vi "main.vi"() -> ()   [LabVIEW 2020]
uses:
  <vilib>/Instr/_visa.llb/VISA Set IO Buffer Mask.ctl
  95f16878-fea6-4ba9-9ba1-5f26283d1fdc.vi
  5cf80d48-7aba-4c71-a3e5-f596ea732e1f.vi
  <vilib>/Instr/_visa.llb/VISA Configure Serial Port (Instr).vi
panel:
  in  "选项卡控件":enum32{"选项卡 1"}(tab)
  in  "?":enum32{"选项卡 1", "选项卡 2"}(tab)
  in  "退出程序":bool
  in  "开始测试":bool
  in  "?":enum32{"Init", "Config"}(tab)
  out "布尔":bool
  in  "打开设备":bool caption="元素入队列"
  in  "Kipcrle":refnum<k15> caption="resource name"
  in  "交流电压输出":dbl caption="Voltage Level"
  in  "输出模式选择":i32(ring) caption="Mode (AC Only)" items=["AC Only", "DC Only", "AC DC"]
  in  "直流偏置":dbl caption="VoltageOffset"
  in  "交流频率":dbl(ring)=50.0 caption="Frequency" items=["50HZ"=50.0, "90HZ"=90.0]
  in  "输出":bool
  in  "电压短时中断测试":bool
  in  "电源适应性测试":bool
  in  "模式选择":enum32{"随机模式"}(tab)
  in  "工作频率随机":bool
  in  "交流电压随机":bool
  in  "短时输出时间随机":bool
  in  "间隔中断时间随机":bool
  in  "关断时间随机":bool
  in  "工作电压":dbl caption="Acv"
  in  "直流偏置编程":dbl caption="Dcv"
  in  "关断电压":dbl caption="Acv"
  in  "upper bound (100)":dbl=100.0 caption="上限(V)"
  in  "lower bound (0)":dbl caption="下限(V)"
  in  "关断电压随机":bool
  in  "中断电压":dbl
  in  "t_off":dbl
  in  "t_gap":dbl
  in  "t_check":dbl
  in  "upper bound (100) 2":dbl=100.0 caption="上限(s)"
  in  "lower bound (0) 2":dbl caption="下限(s)"
  in  "t_on":dbl
  in  "upper bound (100) 3":dbl=100.0 caption="上限(s)"
  in  "lower bound (0) 3":dbl caption="下限(s)"
  in  "间隔中断电压随机":bool
  in  "lower bound (0) 4":dbl caption="下限(s)"
  in  "upper bound (100) 4":dbl=100.0 caption="上限(s)"
  in  "upper bound (100) 5":dbl=100.0 caption="上限(s)"
  in  "lower bound (0) 5":dbl caption="下限(s)"
  in  "工作频率":dbl(ring)=50.0 items=["50Hz"=50.0, "90Hz"=90.0]
  in  "upper bound (100) 6":dbl=100.0 caption="上限(100)"
  in  "lower bound (0) 6":dbl caption="下限(0)"
  in  "lower bound (0) 7":dbl caption="下限(0)"
  in  "upper bound (100) 7":dbl=100.0 caption="上限(100)"
  out "KipcrleErrorOut":errorcluster caption="error out" {"code" format="%.0x"}
  in  "?":enum32{"选项卡 1"}(tab)
  in  "单功能验证":bool
  in  "统一指令集":T1
  in  "设备数量":i8 min=0 max=2
  in  "是否通过串口检测":bool
  in  "?":enum32{"USB", "网口"}(tab)
  in  "VISA资源名称1":refnum<visa-resource-name>
  in  "VISA资源名称":refnum<visa-resource-name>
  in  "stop bits (10: 1 bit)":u16(ring)=10 caption="停止位（10: 1位）" items=["1.0"=10, "1.5"=15, "2.0"=20]
  in  "baud rate (9600)":u32=9600 caption="波特率(9600)"
  in  "parity (0:none)":enum16{"None", "Odd", "Even", "Mark", "Space"}(ring) caption="奇偶（0:无）"
  in  "baud rate (9600) 2":u32=9600 caption="波特率(9600)"
  in  "parity (0:none) 2":enum16{"None", "Odd", "Even", "Mark", "Space"}(ring) caption="奇偶（0:无）"
  in  "stop bits (10: 1 bit) 2":u16(ring)=10 caption="停止位（10: 1位）" items=["1.0"=10, "1.5"=15, "2.0"=20]
  in  "读取的字节":i32=500
  in  "远程端口或服务名称":u16
  in  "地址":string
  in  "发送":bool
  out "码词":string
  in  "自定义输入":string="~\u00010000@SCNTRG1;\u0003"
  in  "等待检测时间(s)":dbl
  out "COM1提示灯":bool
  out "布尔 2":bool
  out "错误输出":errorcluster
  out "模式缓存值":i32(ring) caption="Mode (AC Only)" items=["AC Only", "DC Only", "AC DC"]
  # "AC Source 上位机控制系统  beta v0.1"
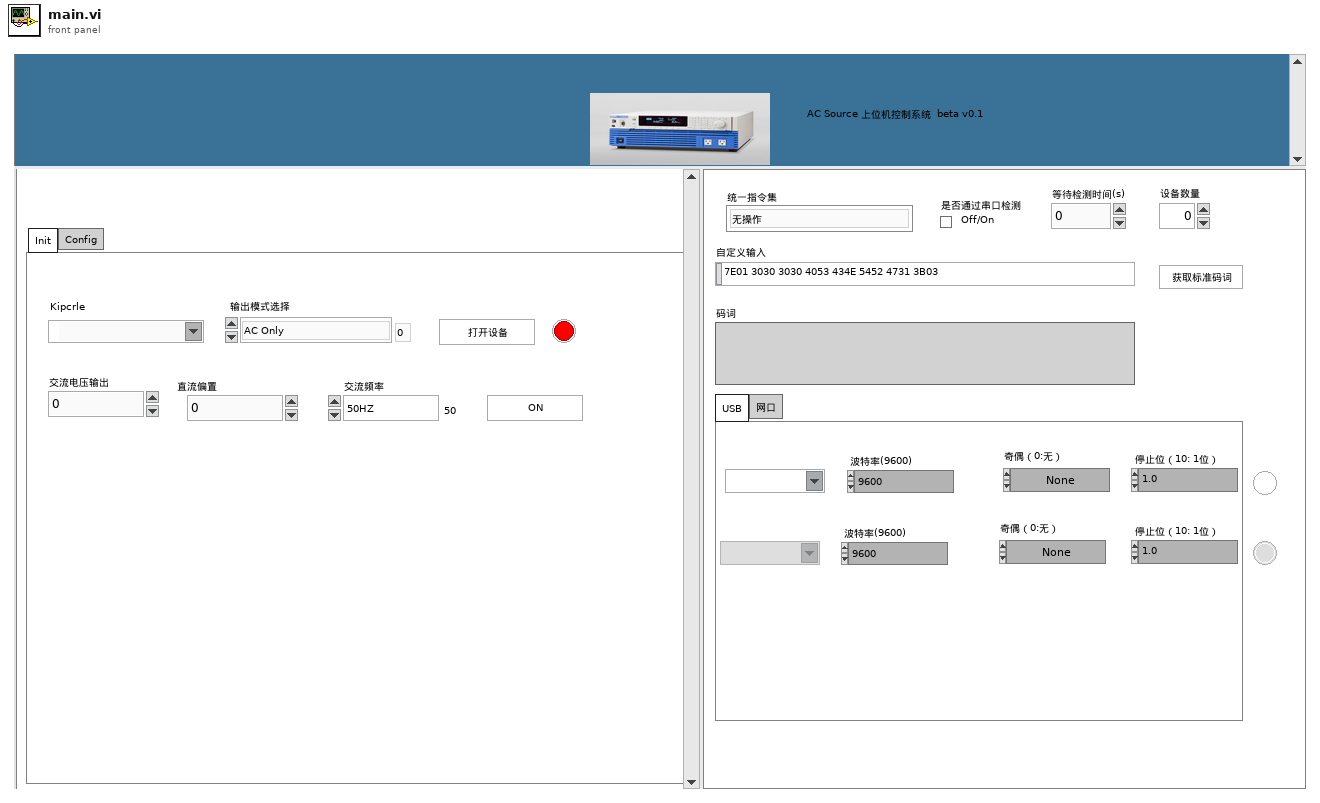
[diagram p1: front panel]
types:
  T1 = typedef "统一指令集.ctl" = enum16{"无操作", "自定义", "波特率切换为9600", "波特率切换为115200", "拍图/解码", "取图", "电平触发模式", "连续读码模式", "睡眠模式", "获取图像分辨率", "开启RTS与CTS流控", "无流控", "感应模式", "红外感应模式", "图像感应模式", "图像与红外感应模式", "切换为串口", "切换为CDC", "关闭照明灯", "开启照明灯", "照明灯常亮", "关闭瞄准灯", "开启瞄准灯", "开启设置码", "连续读码模式2", "触发模式", "0390命令识读模式", "0390连续识读模式", "查询产品序列号", "查询SN空间大小", "产品信息修改开关", "设置产品序列号", "删除序列号", "0390单芯片开启EEPROM写入", "0390单芯片关闭EEPROM写入", "0390单芯片写入产品序列号", "0390单芯片查询产品序列号"}
  T2 = typedef "VISA Set IO Buffer Mask.ctl" = u16
  T3 = enum8{"Enabled", "Disabled", "Disabled and Grayed Out"}
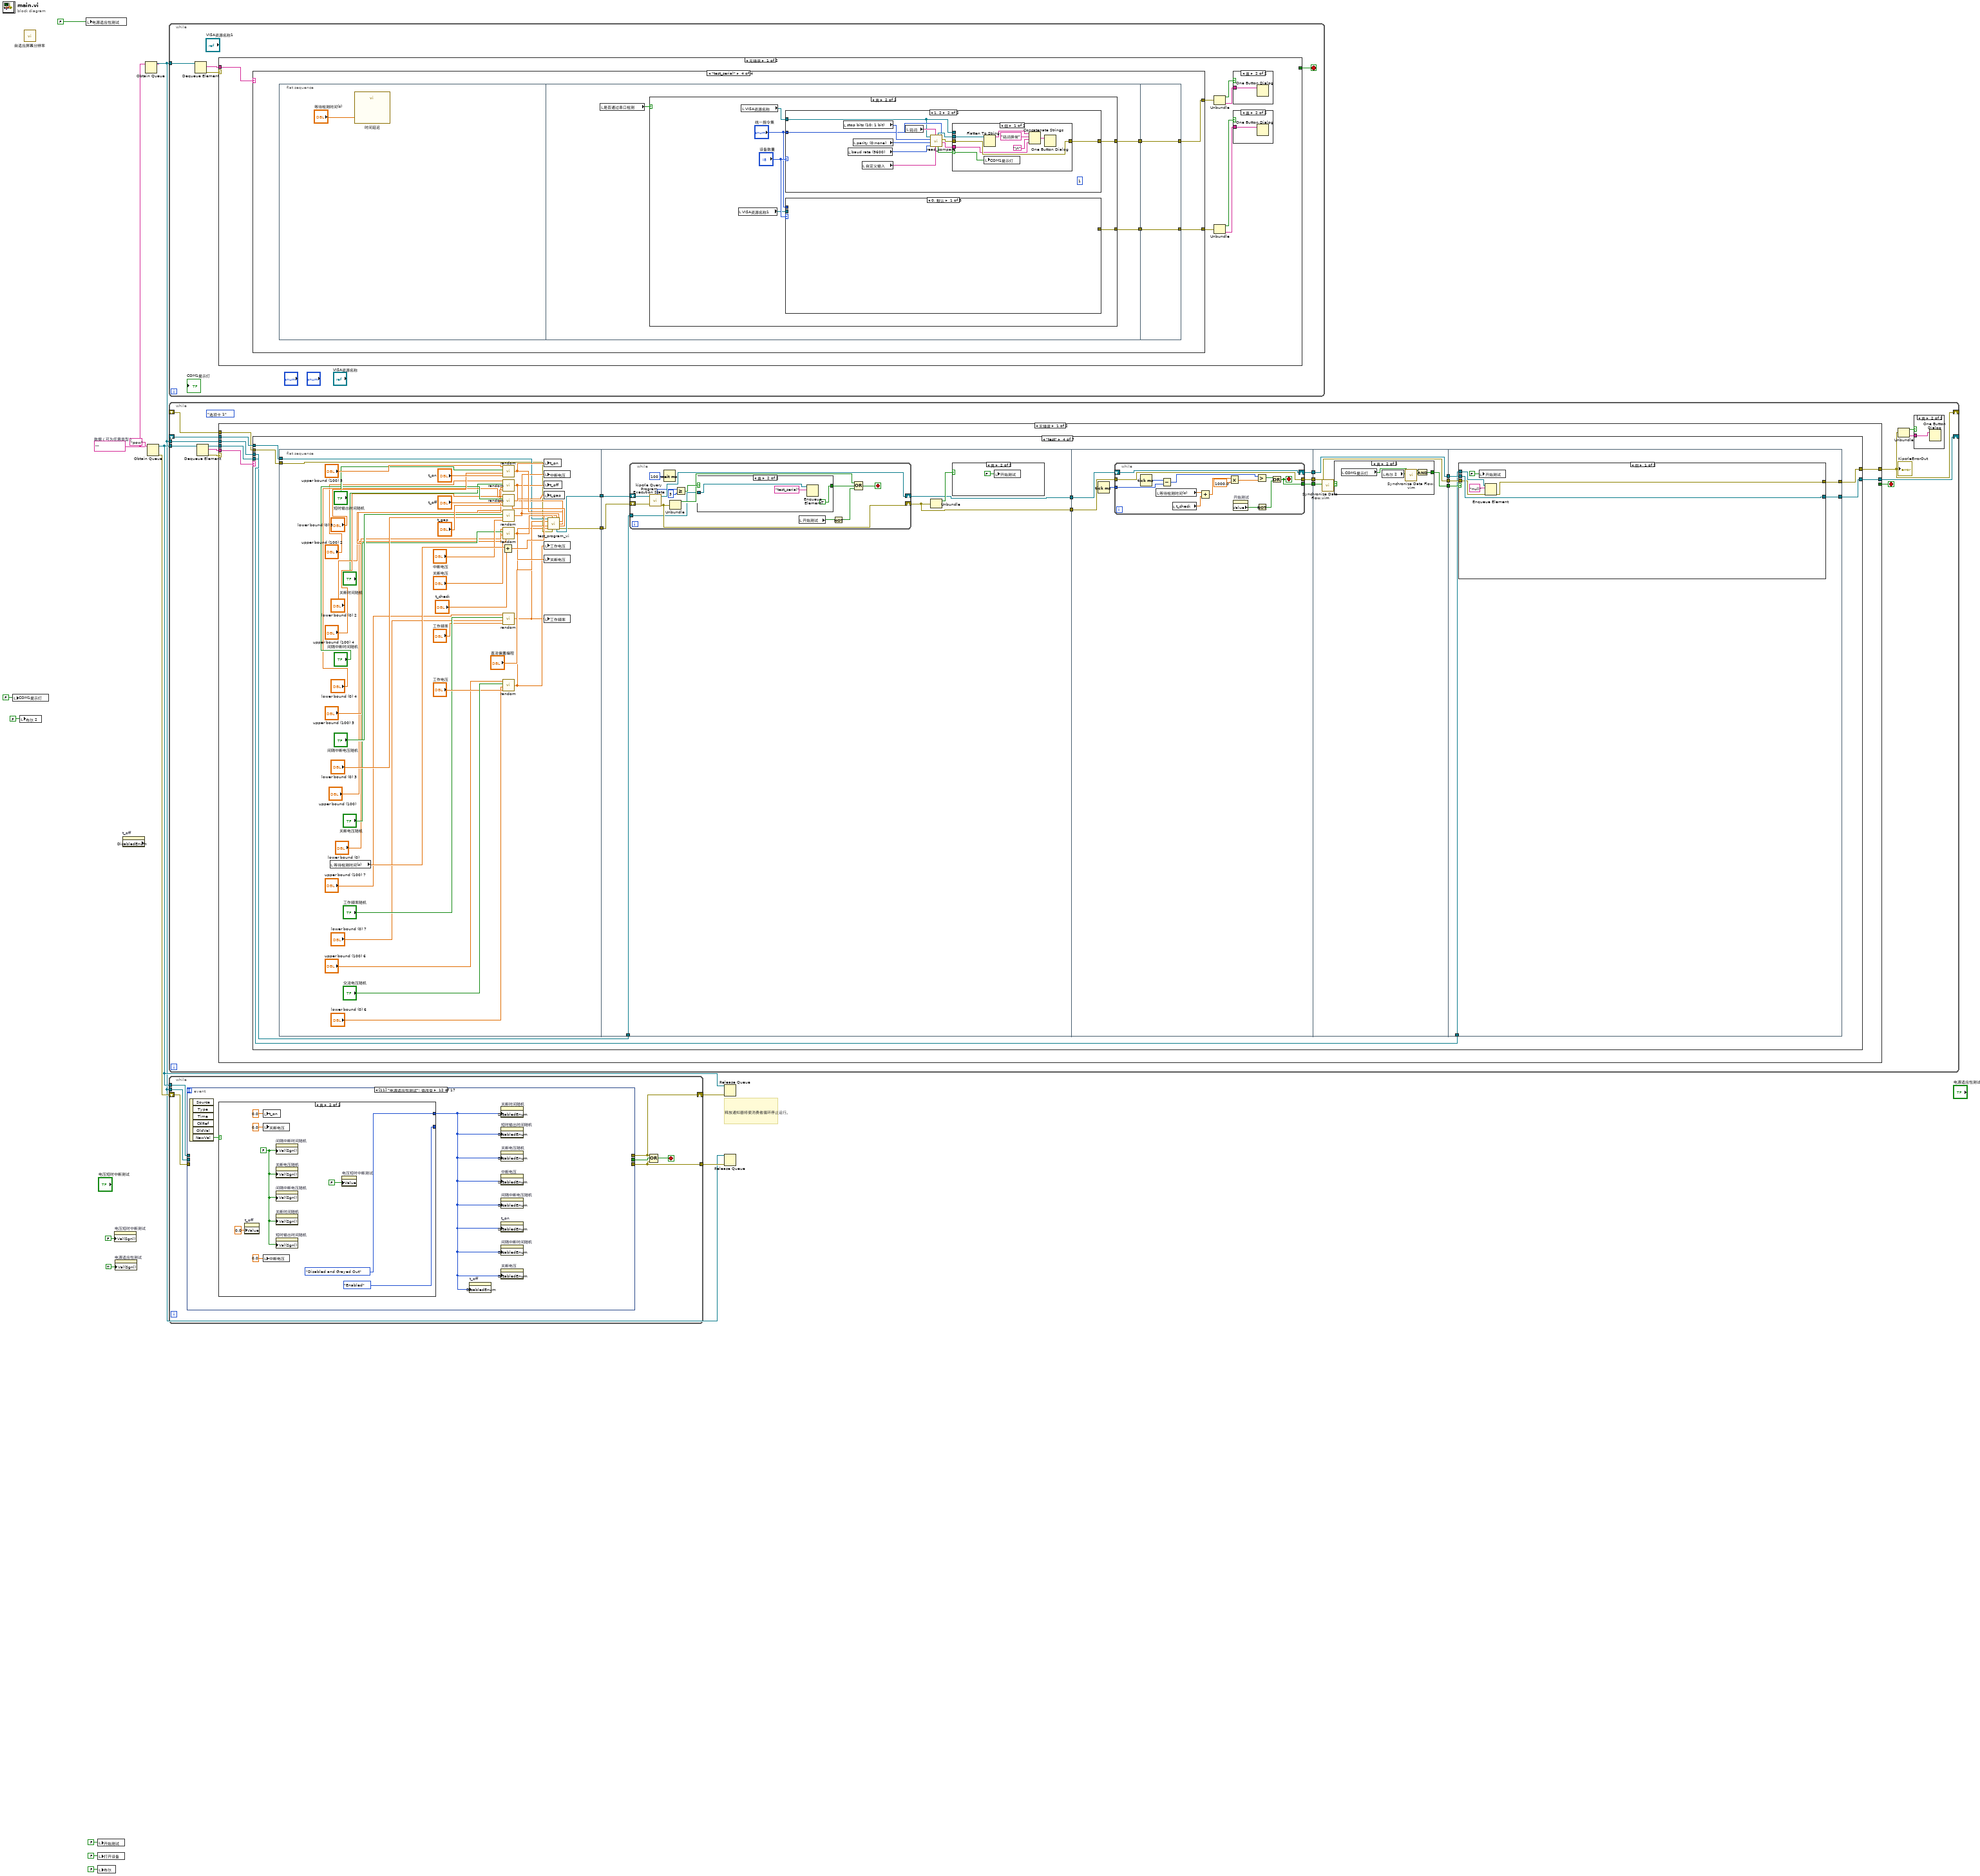
[diagram p0: block diagram]
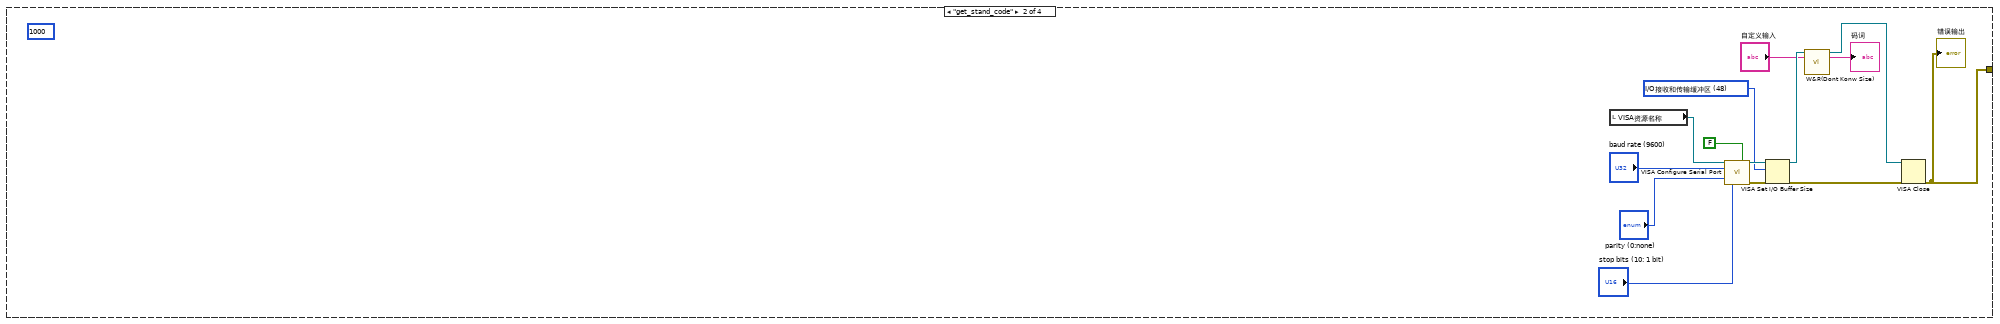
[diagram p5: hidden frame]
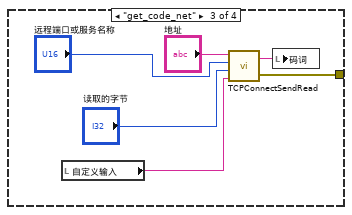
[diagram p6: hidden frame]
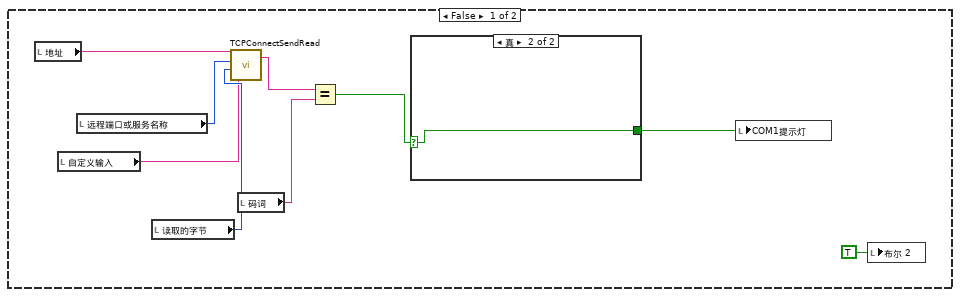
[diagram p7: hidden frame]
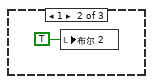
[diagram p9: hidden frame]
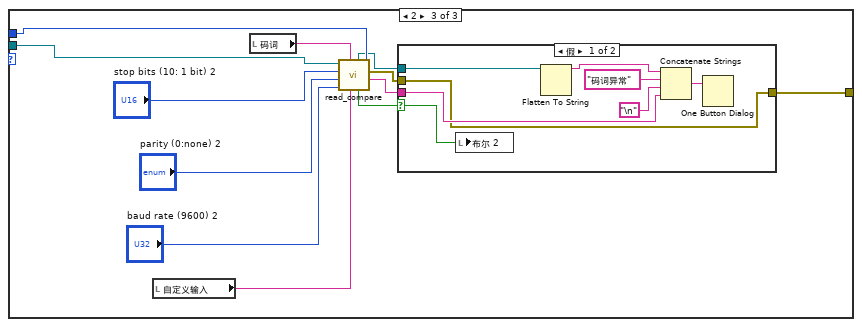
[diagram p10: hidden frame]
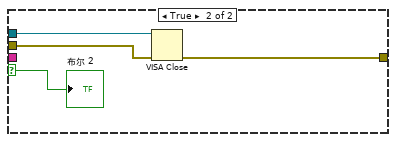
[diagram p11: hidden frame]
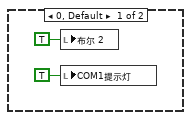
[diagram p12: hidden frame]
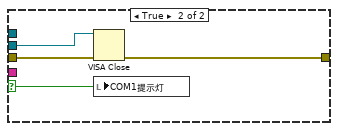
[diagram p13: hidden frame]
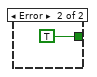
[diagram p14: hidden frame]
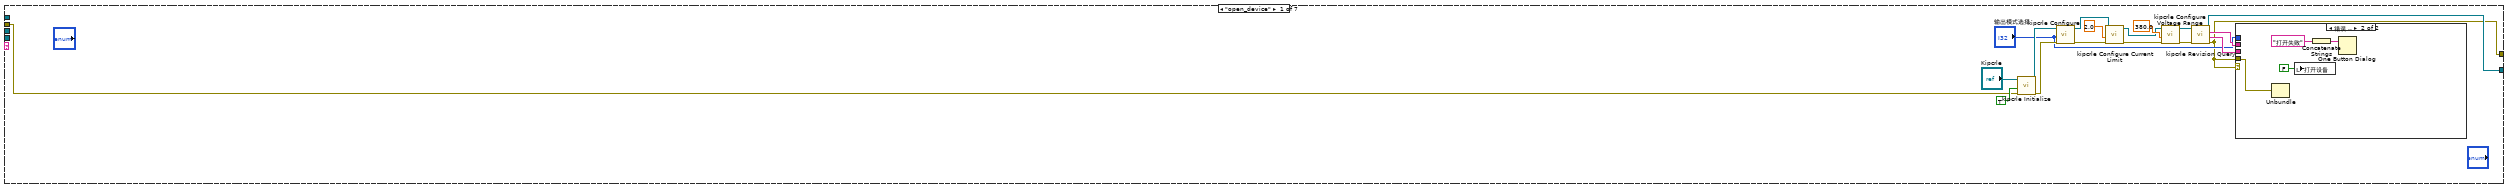
[diagram p16: hidden frame]
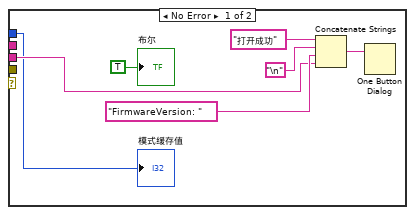
[diagram p17: hidden frame]
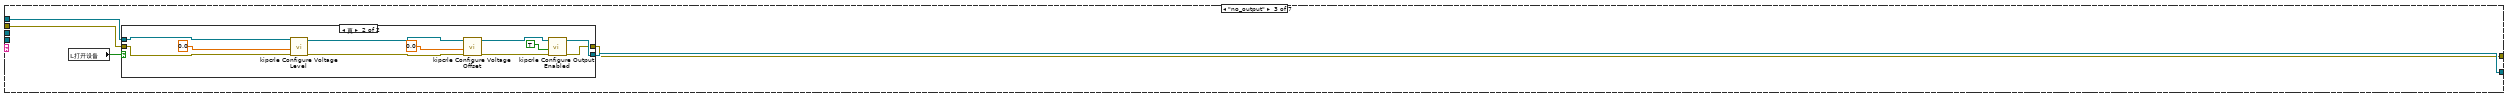
[diagram p19: hidden frame]
diagram:
  w9 = ""  # 数据（可为任意类型）
  # "释放通知器将使消费者循环停止运行。"
  n1 = local write "COM1提示灯"(FALSE ("COM1提示灯")) -> ()
  n2 = local write "布尔 2"(FALSE ("布尔 2")) -> ()
  n3 = call "自适应屏幕分辨率.vi"() -> ()  [unwired: 16 in]
  n4 = local write "电源适应性测试"(FALSE ("电源适应性测试自动分配")) -> ()
  n5 = local write "开始测试"(FALSE ("开始测试")) -> ()
  n6 = local write "打开设备"(FALSE ("打开设备")) -> ()
  n7 = local write "布尔"(FALSE ("布尔")) -> ()
  n8 = property on="电压短时中断测试" class="Bool (严格)"("Val(Sgnl)"=FALSE ("值(信号)")) -> ()  [unwired: 2 in, 2 out]
  n9 = property on="电源适应性测试" class="Bool (严格)"("Val(Sgnl)"=TRUE ("值(信号)")) -> ()  [unwired: 2 in, 2 out]
  n10 = property on="t_off" class="DigNum (严格)" props=["DisabledEnum"]() -> ()  [unwired: 2 in, 3 out]
  n11 = Obtain Queue(element data type=w9) -> (queue out=w6:refnum<queue>)  [unwired: 4 in, 2 out]
  n12 = Obtain Queue(name (unnamed)="pow" ("名称（未命名）"), element data type=w9) -> (queue out=w10:refnum<queue>, error out=w15:errorcluster)  [unwired: 3 in, 1 out]
  n13 = while {
    tunnel: w6 -> [w18]
    stop <- w16 stop-if-true
    n14 = Dequeue Element(queue=w18) -> (element=w17:string, error out=w19:errorcluster)  [unwired: 2 in, 2 out]
    n15 = case shown="无错误" w19 {
      tunnel: w17 -> [w26 _]
      tunnel: [_ TRUE] -> w16
      frame No Error {
        n16 = case shown="\"test_serial\"" w26 {
          tunnel: [_ w38 w45 w52] -> w23
          tunnel: [_ _ _ w51] -> w20
          frame "null ", Default {
          }
          frame "get_stand_code" {
            (unwired) u32 1000 ("字节总数")
            w40 = T2 48 items=["I/O接收缓冲区"=16, "I/O传输缓冲区"=32, "I/O接收和传输缓冲区"=48] ("Mask")
            n17 = local read "VISA资源名称"() -> (w39:refnum<visa-resource-name>)
            n18 = call-poly "VISA Configure Serial Port"("VISA resource name"=w39, "Enable Termination\nChar (T)"=FALSE ("Enable Termination\nChar (T)"), "baud rate (9600)"="baud rate (9600)", "parity (0:none)"="parity (0:none)", "stop bits (10: 1 bit)"="stop bits (10: 1 bit)") -> ("VISA resource name out"=w41:refnum<visa-resource-name>, "error out"=w42:errorcluster)  [unwired: 9 in]
            n19 = VISA Set I/O Buffer Size(VISA resource name=w41, mask (16)=w40, error in (no error)=w42) -> (VISA resource name out=w32:refnum<visa-resource-name>, error out=w33:errorcluster)  [unwired: 1 in]
            n20 = call "W&R(Dont Konw Size).vi"("VISA resource name in"=w32, "写入指令/数据"="自定义输入") -> ("VISA resource name out"=w31:refnum<visa-resource-name>, "读取缓冲区"=→"码词":string)  [unwired: 11 in, 1 out]
            n21 = VISA Close(VISA resource name=w31, error in (no error)=w33) -> (error out=w38:errorcluster)
            "错误输出" <- w38
          }
          frame "get_code_net" {
            n22 = local read "自定义输入"() -> (w43:string)
            n23 = call "TCPConnectSendRead.vi"("数据输入"=w43, "读取的字节"="读取的字节", "远程端口或服务名称"="远程端口或服务名称", "地址"="地址") -> ("错误输出"=w45:errorcluster, "数据输出"=w44:string)
            n24 = local write "码词"(w44) -> ()
          }
          frame "test_serial" {
            n25 = flat-sequence {
              tunnel: [w55] -> w50
              tunnel: [w54] -> w49
              tunnel: [w125] -> w51
              tunnel: [w126] -> w52
              tunnel: w50 -> [w126]
              tunnel: w49 -> [w125]
              frame #0 {
                n26 = call "时间延迟"("Delay Time (s)"="等待检测时间(s)") -> ()  [unwired: 10 in, 1 out]
              }
              frame #1 {
                n27 = local read "是否通过串口检测"() -> (w56:bool)
                n28 = case shown="真" w56 {
                  tunnel: [_ w73] -> w55
                  tunnel: [_ w70] -> w54
                  frame False {
                    n29 = local read "地址"() -> (w64:string)
                    n30 = local read "自定义输入"() -> (w61:string)
                    n31 = local read "远程端口或服务名称"() -> (w63:u16)
                    n32 = local read "读取的字节"() -> (w62:i32)
                    n33 = call "TCPConnectSendRead.vi"("数据输入"=w61, "读取的字节"=w62, "远程端口或服务名称"=w63, "地址"=w64) -> ("数据输出"=w60:string)  [unwired: 1 out]
                    n34 = local read "码词"() -> (w59:string)
                    n35 = Equal?(x=w60, y=w59) -> (x = y?=w58:bool)
                    n36 = case shown="真" w58 {
                      selector: w58 -> [w66 w67]
                      tunnel: [w66 w67] -> w57
                      frame False {
                      }
                      frame True {
                      }
                    }
                    n37 = local write "COM1提示灯"(w57) -> ()
                    n38 = local write "布尔 2"(TRUE ("布尔 2")) -> ()
                  }
                  frame True {
                    n39 = local read "VISA资源名称1"() -> (w69:refnum<visa-resource-name>)
                    n40 = local read "VISA资源名称"() -> (w68:refnum<visa-resource-name>)
                    n41 = case shown="1, 2" "设备数量" {
                      tunnel: [_ w106] -> w73
                      tunnel: "统一指令集" -> [_ w104]
                      tunnel: w68 -> [_ w101]
                      frame 0, Default {
                        n42 = local write "布尔 2"(TRUE ("布尔 2")) -> ()
                        n43 = local write "COM1提示灯"(TRUE ("COM1提示灯")) -> ()
                      }
                      frame 1, 2 {
                        (unwired) i8 1 ("y")
                        n44 = local read "stop bits (10: 1 bit)"() -> (w110:u16)
                        n45 = local read "baud rate (9600)"() -> (w112:u32)
                        n46 = local read "parity (0:none)"() -> (w111:enum16{"None", "Odd", "Even", "Mark", "Space"})
                        n47 = local read "自定义输入"() -> (w109:string)
                        n48 = local read "码词"() -> (w105:string)
                        n49 = call "read_compare.vi"("统一指令集"=w104, "指令"=w109, "应答"=w105, "baud rate (9600)"=w112, "parity (0:none)"=w111, "stop bits (10: 1 bit)"=w110, "VISA resource name"=w101) -> ("码词"=w103:string, "error out"=w107:errorcluster, "布尔"=w102:bool, "VISA resource name out"=w108:refnum<visa-resource-name>)  [unwired: 1 in]
                        n50 = case shown="假" w102 {
                          selector: w102 -> [w113 w121]
                          tunnel: w108 -> [w117 w124]
                          tunnel: w107 -> [w120 w123]
                          tunnel: [w120 w122] -> w106
                          tunnel: w101 -> [_ _]
                          tunnel: w103 -> [w114 _]
                          frame False {
                            n51 = Flatten To String(anything=w117) -> (data string=w116:string)  [unwired: 3 in, 2 out]
                            n52 = local write "COM1提示灯"(w113) -> ()
                            n53 = Concatenate Strings(w116, "码词异常" ("字符串"), "\n", w114) -> (w118:string)
                            n54 = One Button Dialog(message=w118) -> ()  [unwired: 1 in, 1 out]
                          }
                          frame True {
                            n55 = VISA Close(VISA resource name=w124, error in (no error)=w123) -> (error out=w122:errorcluster)
                            n56 = local write "COM1提示灯"(w121) -> ()
                          }
                        }
                      }
                    }
                    n57 = case shown="0, 默认" "设备数量" {
                      tunnel: "统一指令集" -> [_ _ w84]
                      tunnel: [_ _ w78] -> w70
                      tunnel: w69 -> [_ _ w75]
                      frame 0, Default {
                      }
                      frame 1 {
                        n58 = local write "布尔 2"(TRUE ("布尔 2")) -> ()
                      }
                      frame 2 {
                        n59 = local read "自定义输入"() -> (w81:string)
                        n60 = local read "码词"() -> (w82:string)
                        n61 = call "read_compare.vi"("统一指令集"=w84, "指令"=w81, "应答"=w82, "baud rate (9600)"="baud rate (9600) 2", "parity (0:none)"="parity (0:none) 2", "stop bits (10: 1 bit)"="stop bits (10: 1 bit) 2", "VISA resource name"=w75) -> ("码词"=w76:string, "error out"=w77:errorcluster, "布尔"=w80:bool, "VISA resource name out"=w79:refnum<visa-resource-name>)  [unwired: 1 in]
                        n62 = case shown="假" w80 {
                          selector: w80 -> [w87 w95]
                          tunnel: w79 -> [w89 w98]
                          tunnel: [w88 w97] -> w78
                          tunnel: w77 -> [w88 w96]
                          tunnel: w76 -> [w94 _]
                          frame False {
                            n63 = local write "布尔 2"(w87) -> ()
                            n64 = Flatten To String(anything=w89) -> (data string=w91:string)  [unwired: 3 in, 2 out]
                            n65 = Concatenate Strings(w91, "码词异常" ("字符串"), "\n", w94) -> (w92:string)
                            n66 = One Button Dialog(message=w92) -> ()  [unwired: 1 in, 1 out]
                          }
                          frame True {
                            n67 = VISA Close(VISA resource name=w98, error in (no error)=w96) -> (error out=w97:errorcluster)
                            "布尔 2" <- w95
                          }
                        }
                      }
                    }
                  }
                }
              }
              frame #2 {
              }
            }
          }
        }
        n68 = Unbundle(w23) -> ("status"=w24:bool, "source"=w25:string)  [unwired: 1 out]
        n69 = Unbundle(w20) -> ("status"=w22:bool, "source"=w21:string)  [unwired: 1 out]
        n70 = case shown="真" w24 {
          tunnel: w25 -> [_ w28]
          frame False {
          }
          frame True {
            n71 = One Button Dialog(message=w28) -> ()  [unwired: 1 in, 1 out]
          }
        }
        n72 = case shown="真" w22 {
          tunnel: w21 -> [_ w27]
          frame False {
          }
          frame True {
            n73 = One Button Dialog(message=w27) -> ()  [unwired: 1 in, 1 out]
          }
        }
      }
      frame Error {
      }
    }
  }
  n74 = while {
    tunnel: w10 -> [w129]
    shift-right: [w137] -> _
    shift-left: _ -> [w136]
    shift-right: [w134] -> _
    shift-left: _ -> [w135]
    tunnel: w6 -> [w131]
    stop <- w138 stop-if-true
    (unwired) enum32{"选项卡 1"}."选项卡 1"
    n75 = Dequeue Element(queue=w129) -> (queue out=w128:refnum<queue>, element=w130:string, error out=w139:errorcluster)  [unwired: 2 in, 1 out]
    n76 = case shown="无错误" w139 {
      tunnel: w130 -> [w147 _]
      tunnel: [_ TRUE] -> w138
      tunnel: [w146 _] -> w137
      tunnel: [w145 w405] -> w134
      tunnel: w136 -> [w144 w406]
      tunnel: w135 -> [w143 _]
      tunnel: w131 -> [w141 _]
      tunnel: w128 -> [w142 _]
      frame No Error {
        n77 = case shown="\"test\"" w147 {
          tunnel: [w162 _ w178 w203 w355 w378 _] -> w146
          tunnel: [w153 _ w177 w202 w356 w377 w400] -> w145
          tunnel: w144 -> [_ _ w180 w197 w357 w379 w402]
          tunnel: w143 -> [w163 _ w179 w196 w354 w376 w401]
          tunnel: w142 -> [_ _ _ w204 _ _ _]
          tunnel: w141 -> [_ _ _ w195 _ _ _]
          frame "open_device" {
            n78 = call <instrlib>:"kipcrle Initialize.vi"("error in (no error)"=w163, "Reset Device (Off)"=TRUE, "resource name"="Kipcrle") -> ("error out"=w158:errorcluster, "instrument handle out"=w159:refnum<k15>)  [unwired: 7 in]
            n79 = call <instrlib>:"kipcrle Configure.vi"("error in (no error)"=w158, "Mode (AC Only)"="输出模式选择", "instrument handle"=w159) -> ("error out"=w150:errorcluster, "instrument handle out"=w152:refnum<k15>)  [unwired: 4 in, 3 out]
            n80 = call <instrlib>:"kipcrle Configure Current Limit.vi"("error in (no error)"=w150, "Limit"=2.0, "instrument handle"=w152) -> ("error out"=w149:errorcluster, "instrument handle out"=w151:refnum<k15>)  [unwired: 7 in]
            n81 = call <instrlib>:"kipcrle Configure Voltage Range.vi"("error in (no error)"=w149, "Range"=380.0, "instrument handle"=w151) -> ("error out"=w154:errorcluster, "instrument handle out"=w155:refnum<k15>)  [unwired: 7 in]
            n82 = call <instrlib>:"kipcrle Revision Query.vi"("error in (no error)"=w154, "instrument handle"=w155) -> ("error out"=w153:errorcluster, "Firmware Revision"=w160:string, "Instrument Driver Revision"=w161:string, "instrument handle out"=w162:refnum<k15>)  [unwired: 6 in]
            n83 = case shown="错误 .." w153 {
              tunnel: w161 -> [_ _]
              tunnel: w160 -> [w168 _]
              tunnel: "输出模式选择" -> [w167 _]
              tunnel: w153 -> [_ w175]
              frame No Error {
                n84 = Concatenate Strings("打开成功" ("消息"), "\n", "FirmwareVersion: " ("字符串"), w168) -> (w171:string)
                n85 = One Button Dialog(message=w171) -> ()  [unwired: 1 in, 1 out]
                "模式缓存值" <- w167
                "布尔" <- TRUE ("布尔")
              }
              frame Error {
                n86 = Unbundle(w175) -> ()  [unwired: 3 out]
                n87 = local write "打开设备"(FALSE ("打开设备")) -> ()
                n88 = Concatenate Strings("打开失败" ("消息")) -> (w173:string)
                n89 = One Button Dialog(message=w173) -> ()  [unwired: 1 in, 1 out]
              }
            }
          }
          frame "null", Default {
          }
          frame "no_output" {
            n90 = local read "打开设备"() -> (w181:bool)
            n91 = case shown="真" w181 {
              tunnel: w180 -> [w183 w194]
              tunnel: w179 -> [w182 w189]
              tunnel: [w183 w188] -> w178
              tunnel: [w182 w187] -> w177
              frame False {
              }
              frame True {
                n92 = call <instrlib>:"kipcrle Configure Voltage Level.vi"("error in (no error)"=w189, "Voltage Level"=0.0, "instrument handle"=w194) -> ("error out"=w192:errorcluster, "instrument handle out"=w193:refnum<k15>)  [unwired: 7 in]
                n93 = call <instrlib>:"kipcrle Configure Voltage Offset.vi"("error in (no error)"=w192, "VoltageOffset"=0.0, "instrument handle"=w193) -> ("error out"=w190:errorcluster, "instrument handle out"=w191:refnum<k15>)  [unwired: 7 in]
                n94 = call <instrlib>:"kipcrle Configure Output Enabled.vi"("error in (no error)"=w190, "Output Enabled (Off)"=TRUE, "instrument handle"=w191) -> ("error out"=w187:errorcluster, "instrument handle out"=w188:refnum<k15>)  [unwired: 7 in]
              }
            }
          }
          frame "test" {
            n95 = flat-sequence {
              tunnel: [w221] -> w199
              tunnel: [w222] -> w198
              tunnel: w197 -> [w224]
              tunnel: w196 -> [w223]
              tunnel: [w256] -> w201
              tunnel: [w255] -> w200
              tunnel: w199 -> [w258]
              tunnel: w198 -> [w257]
              tunnel: w195 -> [w254]
              tunnel: [w282] -> w210
              tunnel: [w281] -> w209
              tunnel: [w280] -> w208
              tunnel: w201 -> [w284]
              tunnel: w200 -> [w283]
              tunnel: w210 -> [w303]
              tunnel: w209 -> [w302]
              tunnel: w208 -> [w301]
              tunnel: [w303] -> w207
              tunnel: [w302] -> w206
              tunnel: [w299] -> w205
              tunnel: w207 -> [w312]
              tunnel: w206 -> [w313]
              tunnel: w205 -> [w314]
              tunnel: w204 -> [w311]
              tunnel: [w310] -> w203
              tunnel: [w309] -> w202
              frame #0 {
                n96 = local read "等待检测时间(s)"() -> (w251:dbl)
                n97 = Add(x=w251, y="t_check") -> (x+y=w253:dbl)
                n98 = call "random.vi"("输入值"="t_on", "lower bound (0)"="lower bound (0) 5", "布尔"="短时输出时间随机", "upper bound (100)"="upper bound (100) 5") -> ("number"=w250:dbl)
                n99 = call "random.vi"("输入值"="t_off", "lower bound (0)"="lower bound (0) 2", "布尔"="关断时间随机", "upper bound (100)"="upper bound (100) 2") -> ("number"=w235:dbl)
                n100 = call "random.vi"("输入值"="t_gap", "lower bound (0)"="lower bound (0) 4", "布尔"="间隔中断时间随机", "upper bound (100)"="upper bound (100) 4") -> ("number"=w245:dbl)
                n101 = call "random.vi"("输入值"="中断电压", "lower bound (0)"="lower bound (0) 3", "布尔"="间隔中断电压随机", "upper bound (100)"="upper bound (100) 3") -> ("number"=w240:dbl)
                n102 = call "random.vi"("输入值"="关断电压", "lower bound (0)"="lower bound (0)", "布尔"="关断电压随机", "upper bound (100)"="upper bound (100)") -> ("number"=w230:dbl)
                n103 = call "random.vi"("输入值"="工作频率", "lower bound (0)"="lower bound (0) 7", "布尔"="工作频率随机", "upper bound (100)"="upper bound (100) 7") -> ("number"=w211:dbl)
                n104 = call "random.vi"("输入值"="工作电压", "lower bound (0)"="lower bound (0) 6", "布尔"="交流电压随机", "upper bound (100)"="upper bound (100) 6") -> ("number"=w216:dbl)
                n105 = local write "t_on"(w250) -> ()
                n106 = local write "中断电压"(w240) -> ()
                n107 = local write "t_off"(w235) -> ()
                n108 = local write "t_gap"(w245) -> ()
                n109 = local write "工作电压"(w216) -> ()
                n110 = local write "关断电压"(w230) -> ()
                n111 = local write "工作频率"(w211) -> ()
                n112 = call "test_program_vi.vi"("instrument handle"=w224, "t_check"=w253, "关断电压"=w230, "中断电压"=w240, "工作频率"=w211, "t_on"=w250, "t_off"=w235, "直流偏置"="直流偏置编程", "t_gap"=w245, "工作电压"=w216, "error in (no error)"=w223) -> ("instrument handle out"=w222:refnum<k15>, "error out"=w221:errorcluster)  [unwired: 3 in]
              }
              frame #1 {
                n113 = while {
                  shift-right: [w264] -> w256
                  shift-left: w258 -> [w272]
                  shift-right: [w273] -> w255
                  shift-left: w257 -> [w274]
                  tunnel: w254 -> [w261]
                  stop <- w267 stop-if-true
                  n114 = call <instrlib>:"kipcrle Query Program Execution State.vi"("error in (no error)"=w272, "instrument handle"=w274) -> ("error out"=w264:errorcluster, "instrument handle out"=w273:refnum<k15>, "StepNo"=w271:i32)  [unwired: 4 in, 3 out]
                  n115 = Wait (ms)(milliseconds to wait=u32 100 ("等待时间（毫秒）")) -> ()  [unwired: 1 out]
                  n116 = Unbundle(w264) -> ("status"=w263:bool)  [unwired: 2 out]
                  n117 = Greater Or Equal?(x=w271, y=3) -> (x >= y?=w269:bool)
                  n118 = case shown="真" w269 {
                    tunnel: [FALSE TRUE] -> w268
                    tunnel: w261 -> [_ w276]
                    frame False {
                    }
                    frame True {
                      n119 = Enqueue Element(queue=w276, element="test_serial" ("元素")) -> ()  [unwired: 2 in, 3 out]
                    }
                  }
                  n120 = local read "开始测试"() -> (w266:bool)
                  n121 = Not(x=w266) -> (.not. x?=w265:bool)
                  n122 = Compound Arithmetic op=OR ("复合运算")(w263, w268, w265) -> (w267:bool)
                }
                n123 = Unbundle(w256) -> ("status"=w259:bool)  [unwired: 2 out]
                n124 = case shown="真" w259 {
                  frame False {
                  }
                  frame True {
                    n125 = local write "开始测试"(FALSE ("开始测试")) -> ()
                  }
                }
              }
              frame #2 {
                n126 = Tick Count (ms)() -> (millisecond timer value=w279:u32)
                n127 = while {
                  tunnel: [w297] -> w282
                  tunnel: w284 -> [w297]
                  shift-right: [w298] -> w281
                  shift-left: w283 -> [w298]
                  tunnel: w279 -> [w293]
                  tunnel: [w285] -> w280
                  stop <- w285 stop-if-true
                  n128 = Tick Count (ms)() -> (millisecond timer value=w294:u32)
                  n129 = local read "等待检测时间(s)"() -> (w291:dbl)
                  n130 = Subtract(x=w294, y=w293) -> (x-y=w292:u32)
                  n131 = local read "t_check"() -> (w290:dbl)
                  n132 = Add(x=w291, y=w290) -> (x+y=w289:dbl)
                  n133 = Multiply(x=w289, y=1000.0) -> (x*y=w287:dbl)
                  n134 = property on="开始测试" class="Bool (严格)"() -> ("Value"=w296:bool)  [unwired: 2 in, 2 out]
                  n135 = Greater?(x=w292, y=w287) -> (0:w286:bool)
                  n136 = Not(x=w296) -> (.not. x?=w295:bool)
                  n137 = Or(x=w286, y=w295) -> (x .or. y?=w285:bool)
                }
              }
              frame #3 {
                n138 = call "Synchronize Data Flow.vim"("input 2"=w301) -> ("output 2"=w300:bool)  [unwired: 3 in, 3 out]
                n139 = case shown="真" w300 {
                  tunnel: [_ w308] -> w299
                  frame False {
                  }
                  frame True {
                    n140 = local read "COM1提示灯"() -> (w307:bool)
                    n141 = local read "布尔 2"() -> (w306:bool)
                    n142 = call "Synchronize Data Flow.vim"("input 2"=w306, "input 1"=w307) -> ("output 2"=w304:bool, "output 1"=w305:bool)  [unwired: 2 in, 2 out]
                    n143 = And(x=w305, y=w304) -> (x .and. y?=w308:bool)
                  }
                }
              }
              frame #4 {
                n144 = case shown="假" w314 {
                  tunnel: [w320 w323] -> w310
                  tunnel: w313 -> [w320 w324]
                  tunnel: w312 -> [w318 w322]
                  tunnel: [w317 w325] -> w309
                  tunnel: w311 -> [w316 w326]
                  frame False {
                    n145 = local write "开始测试"(FALSE ("开始测试")) -> ()
                    n146 = Enqueue Element(queue=w316, element="null" ("元素"), error in (no error)=w318) -> (error out=w317:errorcluster)  [unwired: 1 in, 2 out]
                  }
                  frame True {
                    n147 = local read "开始测试"() -> (w327:bool)
                    n148 = case shown="真" w327 {
                      tunnel: ["null" ("元素") w334] -> w328
                      tunnel: w324 -> [_ w335]
                      tunnel: [_ w333] -> w323
                      tunnel: w322 -> [_ w331]
                      tunnel: [_ w330] -> w321
                      frame False {
                      }
                      frame True {
                        n149 = flat-sequence {
                          tunnel: w335 -> [w339]
                          tunnel: [w338] -> w332
                          tunnel: w331 -> [w337]
                          tunnel: [w336] -> w330
                          tunnel: ["test" ("元素")] -> w334
                          tunnel: [w348] -> w333
                          tunnel: w332 -> [w348]
                          frame #0 {
                            n150 = while {
                              tunnel: w339 -> [w347]
                              tunnel: [w342] -> w338
                              tunnel: w337 -> [w341]
                              tunnel: [w340] -> w336
                              stop <- w344 stop-if-true
                              n151 = call <instrlib>:"kipcrle Query Program Execution State.vi"("error in (no error)"=w341, "instrument handle"=w347) -> ("error out"=w340:errorcluster, "State"=w346:i32, "instrument handle out"=w342:refnum<k15>)  [unwired: 4 in, 3 out]
                              n152 = Wait (ms)(milliseconds to wait=u32 100 ("等待时间（毫秒）")) -> ()  [unwired: 1 out]
                              n153 = Equal?(x=w346, y=0) -> (x = y?=w344:bool)
                            }
                          }
                          frame #1 {
                            n154 = local write "COM1提示灯"(FALSE ("COM1提示灯")) -> ()
                            n155 = local write "布尔 2"(FALSE ("布尔 2")) -> ()
                          }
                        }
                      }
                    }
                    n156 = Enqueue Element(queue=w326, element=w328, error in (no error)=w321) -> (error out=w325:errorcluster)  [unwired: 1 in, 2 out]
                  }
                }
              }
            }
          }
          frame "mode_select" {
            # "选择更改模式，当当前的值有输出时，ACDC 模式下有配置，无法配置 ,需要reset device"
            n157 = local read "打开设备"() -> (w352:bool)
            n158 = case shown="假" w352 {
              tunnel: [FALSE ("T button?") w359] -> w353
              frame False {
              }
              frame True {
                n159 = Two Button Dialog(message="这将会导致丢失当前的状态是否更改" ("消息")) -> (T button?=w359:bool)  [unwired: 2 in]
              }
            }
            n160 = case shown="真" w353 {
              tunnel: w357 -> [_ w369]
              tunnel: [_ w371] -> w356
              tunnel: [_ w370] -> w355
              tunnel: w354 -> [_ w368]
              tunnel: w352 -> [w361 _]
              frame False {
                n161 = case shown="真" w361 {
                  frame False {
                  }
                  frame True {
                    # "用于不打开的设备的情况，选择又不改当前的模式了"
                    n162 = local read "模式缓存值"() -> (w362:i32)
                    n163 = local write "输出模式选择"(w362) -> ()
                  }
                }
              }
              frame True {
                n164 = call <instrlib>:"kipcrle Reset.vi"("error in (no error)"=w368, "instrument handle"=w369) -> ("error out"=w367:errorcluster, "instrument handle out"=w365:refnum<k15>)  [unwired: 8 in]
                n165 = call <instrlib>:"kipcrle Configure Voltage Range.vi"("Range"=380.0, "instrument handle"=w365) -> ("instrument handle out"=w364:refnum<k15>)  [unwired: 8 in, 1 out]
                n166 = local read "输出模式选择"() -> (w366:i32)
                n167 = local write "模式缓存值"(w366) -> ()
                n168 = call <instrlib>:"kipcrle Configure Coupling Mode.vi"("error in (no error)"=w367, "Mode (AC)"=w366, "instrument handle"=w364) -> ("error out"=w371:errorcluster, "instrument handle out"=w370:refnum<k15>)  [unwired: 7 in]
              }
            }
          }
          frame "output" {
            n169 = Greater?(x="交流电压输出", y=20.0) -> (0:w373:bool)
            n170 = case shown="假" w373 {
              tunnel: [TRUE ("T button?") w382] -> w372
              frame False {
              }
              frame True {
                n171 = Two Button Dialog(message="该电压超过安全电压是否输出" ("消息")) -> (T button?=w382:bool)  [unwired: 2 in]
              }
            }
            n172 = case shown="真" w372 {
              tunnel: w379 -> [w385 w397]
              tunnel: [w385 w391] -> w378
              tunnel: [w384 w389] -> w377
              tunnel: w376 -> [w384 w387]
              tunnel: "交流电压输出" -> [_ w386]
              frame False {
                n173 = local write "输出"(FALSE ("输出")) -> ()
              }
              frame True {
                n174 = call <instrlib>:"kipcrle Configure Output Enabled.vi"("error in (no error)"=w387, "Output Enabled (Off)"=TRUE, "instrument handle"=w397) -> ("error out"=w399:errorcluster, "instrument handle out"=w398:refnum<k15>)  [unwired: 7 in]
                n175 = call <instrlib>:"kipcrle Configure Voltage Level.vi"("error in (no error)"=w399, "Voltage Level"=w386, "instrument handle"=w398) -> ("error out"=w394:errorcluster, "instrument handle out"=w395:refnum<k15>)  [unwired: 7 in]
                n176 = call <instrlib>:"kipcrle Configure Voltage Offset.vi"("error in (no error)"=w394, "VoltageOffset"="直流偏置", "instrument handle"=w395) -> ("error out"=w390:errorcluster, "instrument handle out"=w392:refnum<k15>)  [unwired: 7 in]
                n177 = call <instrlib>:"kipcrle Configure Frequency.vi"("error in (no error)"=w390, "Frequency"="交流频率", "instrument handle"=w392) -> ("error out"=w389:errorcluster, "instrument handle out"=w391:refnum<k15>)  [unwired: 7 in]
              }
            }
          }
          frame "close_dev" {
            n178 = call <instrlib>:"kipcrle Close.vi"("error in (no error)"=w401, "instrument handle"=w402) -> ("error out"=w400:errorcluster)  [unwired: 9 in]
            n179 = case shown="错误 .." w400 {
              frame No Error {
                n180 = local write "布尔"(FALSE ("布尔")) -> ()
              }
              frame Error {
              }
            }
          }
        }
      }
      frame Error {
        # "对任意分支返回真，使循环停止运行。"
        n181 = local read "打开设备"() -> (w404:bool)
        n182 = case shown="真" w404 {
          tunnel: w406 -> [_ w409]
          tunnel: [_ w408] -> w405
          frame False {
          }
          frame True {
            n183 = call <instrlib>:"kipcrle Close.vi"("instrument handle"=w409) -> ("error out"=w408:errorcluster)  [unwired: 10 in]
          }
        }
      }
    }
    "KipcrleErrorOut" <- w134
    n184 = Unbundle(w134) -> ("status"=w133:bool, "source"=w132:string)  [unwired: 1 out]
    n185 = case shown="真" w133 {
      tunnel: w132 -> [_ w140]
      frame False {
      }
      frame True {
        n186 = One Button Dialog(message=w140) -> ()  [unwired: 1 in, 1 out]
      }
    }
  }
  n187 = while {
    shift-right: [w412] -> w8
    shift-left: w15 -> [w415]
    tunnel: w10 -> [w416]
    tunnel: w6 -> [w411]
    tunnel: [w410] -> w7
    stop <- w413 stop-if-true
    n188 = event shown="[11] \"电源适应性测试\": 值改变" {
      selector: _ -> [_ _ _ _ _ _ _ _ _ _ _ _ _ _ _ _ _]
      dyn-events: _ -> [_ _ _ _ _ _ _ _ _ _ _ _ _ _ _ _ _]
      timeout: _ -> [_ _ _ _ _ _ _ _ _ _ _ _ _ _ _ _ _]
      tunnel: w416 -> [w421 w426 w434 _ _ _ _ _ _ _ _ _ _ _ w494 _ _]
      tunnel: w415 -> [w420 _ w433 _ _ _ _ _ _ w462 _ _ _ _ _ _ _]
      tunnel: [w419 w427 w432 _ _ _ _ _ _ w462 _ _ _ _ w495 _ _] -> w412
      tunnel: [_ _ _ _ _ _ _ _ _ "退出程序" _ _ _ _ _ TRUE ("退出程序") TRUE ("退出程序")] -> w414
      tunnel: w411 -> [_ _ _ _ _ _ w452 w456 _ _ _ _ _ _ _ _ _]
      tunnel: [_ _ _ _ _ _ w451 _ _ _ _ _ _ _ _ _ _] -> w410
      event "打开设备": Value Change {
        n189 = event-data() -> ()  [unwired: 1 in, 1 out]
        n190 = case shown="真" "打开设备" {
          tunnel: ["close_dev" ("element") "open_device" ("element")] -> w417
          frame False {
          }
          frame True {
          }
        }
        n191 = Enqueue Element(queue=w421, element=w417, error in (no error)=w420) -> (error out=w419:errorcluster)  [unwired: 1 in, 2 out]
      }
      event "输出": Value Change {
        n192 = event-data() -> ("NewVal"=w424:bool)  [unwired: 1 in, 2 out]
        n193 = case shown="假" w424 {
          tunnel: ["no_output" ("元素") "output" ("元素")] -> w425
          frame False {
          }
          frame True {
          }
        }
        n194 = Enqueue Element(queue=w426, element=w425) -> (error out=w427:errorcluster)  [unwired: 2 in, 2 out]
      }
      event "开始测试": Value Change {
        n195 = event-data() -> ("NewVal"=w430:bool)  [unwired: 1 in, 3 out]
        n196 = case shown="真" w430 {
          tunnel: ["" ("元素") "test" ("元素")] -> w431
          frame False {
          }
          frame True {
          }
        }
        n197 = Enqueue Element(queue=w434, element=w431, error in (no error)=w433) -> (error out=w432:errorcluster)  [unwired: 1 in, 2 out]
      }
      event "间隔中断电压随机": Value Change {
        n198 = event-data() -> ("NewVal"=w438:bool)  [unwired: 1 in, 5 out]
        n199 = case shown="假" w438 {
          tunnel: [T3."Disabled and Grayed Out" ("禁用") T3."Enabled" ("禁用")] -> w437
          frame False {
          }
          frame True {
          }
        }
        n200 = property on="upper bound (100) 3" class="DigNum (严格)"("DisabledEnum"=w437) -> ()  [unwired: 2 in, 2 out]
        n201 = property on="lower bound (0) 3" class="DigNum (严格)"("DisabledEnum"=w437) -> ()  [unwired: 2 in, 2 out]
      }
      event "间隔中断时间随机": Value Change {
        n202 = event-data() -> ("NewVal"=w442:bool)  [unwired: 1 in, 5 out]
        n203 = case shown="假" w442 {
          tunnel: [T3."Disabled and Grayed Out" ("禁用") T3."Enabled" ("禁用")] -> w441
          frame False {
          }
          frame True {
          }
        }
        n204 = property on="lower bound (0) 4" class="DigNum (严格)"("DisabledEnum"=w441) -> ()  [unwired: 2 in, 2 out]
        n205 = property on="upper bound (100) 4" class="DigNum (严格)"("DisabledEnum"=w441) -> ()  [unwired: 2 in, 2 out]
      }
      event "短时输出时间随机": Value Change {
        n206 = event-data() -> ("NewVal"=w446:bool)  [unwired: 1 in, 5 out]
        n207 = case shown="假" w446 {
          tunnel: [T3."Disabled and Grayed Out" ("禁用") T3."Enabled" ("禁用")] -> w445
          frame False {
          }
          frame True {
          }
        }
        n208 = property on="lower bound (0) 5" class="DigNum (严格)"("DisabledEnum"=w445) -> ()  [unwired: 2 in, 2 out]
        n209 = property on="upper bound (100) 5" class="DigNum (严格)"("DisabledEnum"=w445) -> ()  [unwired: 2 in, 2 out]
      }
      event "发送": Value Change {
        n210 = event-data() -> ()  [unwired: 1 in, 6 out]
        n211 = local read "是否通过串口检测"() -> (w450:bool)
        n212 = case shown="真" w450 {
          tunnel: ["get_code_net" ("元素") "get_stand_code" ("元素")] -> w449
          frame False {
          }
          frame True {
          }
        }
        n213 = Enqueue Element(queue=w452, element=w449) -> (error out=w451:errorcluster)  [unwired: 2 in, 2 out]
      }
      event "单功能验证": Value Change {
        n214 = event-data() -> ()  [unwired: 1 in, 6 out]
        n215 = Enqueue Element(queue=w456, element="test" ("元素")) -> ()  [unwired: 2 in, 3 out]
      }
      event "关断时间随机": Value Change {
        n216 = event-data() -> ("NewVal"=w458:bool)  [unwired: 1 in, 3 out]
        n217 = case shown="假" w458 {
          tunnel: [T3."Disabled and Grayed Out" ("禁用") T3."Enabled" ("禁用")] -> w457
          frame False {
          }
          frame True {
          }
        }
        n218 = property on="upper bound (100) 2" class="DigNum (严格)"("DisabledEnum"=w457) -> ()  [unwired: 2 in, 2 out]
        n219 = property on="lower bound (0) 2" class="DigNum (严格)"("DisabledEnum"=w457) -> ()  [unwired: 2 in, 2 out]
      }
      event "退出程序": Value Change {
        n220 = event-data() -> ()  [unwired: 1 in, 1 out]
        n221 = local write "开始测试"(FALSE ("开始测试")) -> ()
      }
      event "设备数量": Value Change {
        n222 = event-data() -> ("NewVal"=w468:i8)  [unwired: 1 in, 5 out]
        n223 = case shown="2" w468 {
          tunnel: [w469 w470 w471] -> w467
          tunnel: [w469 w470 w472] -> w466
          tunnel: [w469 w470 w471] -> w465
          tunnel: [w469 w470 w472] -> w464
          frame 0, Default {
            w469 = T3."Disabled and Grayed Out" ("禁用")
          }
          frame 2 {
            w470 = T3."Enabled" ("禁用")
          }
          frame 1 {
            w471 = T3."Disabled and Grayed Out" ("禁用")
            w472 = T3."Enabled" ("禁用")
          }
        }
        n224 = property on="VISA资源名称" class="VISAName"("DisabledEnum"=w464) -> ()  [unwired: 2 in, 2 out]
        n225 = property on="布尔 2" class="Bool (严格)"("DisabledEnum"=w465) -> ()  [unwired: 2 in, 2 out]
        n226 = property on="COM1提示灯" class="Bool (严格)"("DisabledEnum"=w466) -> ()  [unwired: 2 in, 2 out]
        n227 = property on="VISA资源名称1" class="VISAName"("DisabledEnum"=w467) -> ()  [unwired: 2 in, 2 out]
      }
      event "电源适应性测试": Value Change {
        n228 = event-data() -> ("NewVal"=w474:bool)  [unwired: 1 in, 5 out]
        n229 = case shown="真" w474 {
          tunnel: [T3."Disabled and Grayed Out" ("禁用") T3."Enabled" ("禁用")] -> _
          tunnel: [T3."Enabled" ("禁用") T3."Disabled and Grayed Out" ("禁用")] -> w473
          frame False {
          }
          frame True {
            w479 = FALSE ("关断电压随机")
            n230 = property on="t_off" class="DigNum (严格)"("Value"=0.0 ("t_off")) -> ()  [unwired: 2 in, 2 out]
            n231 = local write "t_on"(0.0 ("t_on")) -> ()
            n232 = local write "关断电压"(0.0 ("关断电压")) -> ()
            n233 = local write "中断电压"(0.0 ("中断电压")) -> ()
            n234 = property on="间隔中断时间随机" class="Bool (严格)"("Val(Sgnl)"=w479) -> ()  [unwired: 2 in, 2 out]
            n235 = property on="关断电压随机" class="Bool (严格)"("Val(Sgnl)"=w479) -> ()  [unwired: 2 in, 2 out]
            n236 = property on="间隔中断电压随机" class="Bool (严格)"("Val(Sgnl)"=w479) -> ()  [unwired: 2 in, 2 out]
            n237 = property on="关断时间随机" class="Bool (严格)"("Val(Sgnl)"=w479) -> ()  [unwired: 2 in, 2 out]
            n238 = property on="短时输出时间随机" class="Bool (严格)"("Val(Sgnl)"=w479) -> ()  [unwired: 2 in, 2 out]
            n239 = property on="电压短时中断测试" class="Bool (严格)"("Value"=FALSE ("值(信号)")) -> ()  [unwired: 2 in, 2 out]
          }
        }
        n240 = property on="t_off" class="DigNum (严格)"("DisabledEnum"=w473) -> ()  [unwired: 2 in, 2 out]
        n241 = property on="关断时间随机" class="Bool (严格)"("DisabledEnum"=w473) -> ()  [unwired: 2 in, 2 out]
        n242 = property on="短时输出时间随机" class="Bool (严格)"("DisabledEnum"=w473) -> ()  [unwired: 2 in, 2 out]
        n243 = property on="关断电压随机" class="Bool (严格)"("DisabledEnum"=w473) -> ()  [unwired: 2 in, 2 out]
        n244 = property on="中断电压" class="DigNum (严格)"("DisabledEnum"=w473) -> ()  [unwired: 2 in, 2 out]
        n245 = property on="间隔中断电压随机" class="Bool (严格)"("DisabledEnum"=w473) -> ()  [unwired: 2 in, 2 out]
        n246 = property on="t_on" class="DigNum (严格)"("DisabledEnum"=w473) -> ()  [unwired: 2 in, 2 out]
        n247 = property on="间隔中断时间随机" class="Bool (严格)"("DisabledEnum"=w473) -> ()  [unwired: 2 in, 2 out]
        n248 = property on="关断电压" class="DigNum (严格)"("DisabledEnum"=w473) -> ()  [unwired: 2 in, 2 out]
      }
      event "电压短时中断测试": Value Change {
        n249 = event-data() -> ("NewVal"=w486:bool)  [unwired: 1 in, 5 out]
        n250 = case shown="真" w486 {
          tunnel: [TRUE ("值(信号)") FALSE ("值(信号)")] -> w485
          frame False {
          }
          frame True {
          }
        }
        n251 = property on="电源适应性测试" class="Bool (严格)"("Val(Sgnl)"=w485) -> ()  [unwired: 2 in, 2 out]
      }
      event "关断电压随机": Value Change {
        n252 = event-data() -> ("NewVal"=w490:bool)  [unwired: 1 in, 3 out]
        n253 = case shown="假" w490 {
          tunnel: [T3."Disabled and Grayed Out" ("禁用") T3."Enabled" ("禁用")] -> w489
          frame False {
          }
          frame True {
          }
        }
        n254 = property on="lower bound (0)" class="DigNum (严格)"("DisabledEnum"=w489) -> ()  [unwired: 2 in, 2 out]
        n255 = property on="upper bound (100)" class="DigNum (严格)"("DisabledEnum"=w489) -> ()  [unwired: 2 in, 2 out]
      }
      event "输出模式选择": Value Change {
        n256 = event-data() -> ()  [unwired: 1 in, 3 out]
        n257 = Enqueue Element(queue=w494, element="mode_select" ("元素")) -> (error out=w495:errorcluster)  [unwired: 2 in, 2 out]
      }
      event Application Instance Close {
        n258 = event-data() -> ()  [unwired: 1 in, 3 out]
      }
      event Panel Close {
        n259 = event-data() -> ()  [unwired: 1 in, 3 out]
      }
    }
    n260 = Compound Arithmetic op=OR ("复合运算")(w412, w414, w410) -> (w413:bool)
  }
  n261 = Release Queue(queue=w10, error in (no error)=w8) -> ()  [unwired: 1 in, 3 out]
  n262 = Release Queue(queue=w6, error in (no error)=w7) -> ()  [unwired: 1 in, 3 out]
